vi "Tree Map from Pretty XML.vi"(7 "Parent Path (empty)":string, 10 "Pretty XML":string, 11 "Tree Map In (empty)":T1) -> (0 "Path Invalid":bool, 3 "Tree Map Out":T1)   [LabVIEW 2020, in "Tree Map.lvlib"]
doc: "Unflattens an XML string following the Tree Map API definition. This VI does not work with standard inbuilt LabVIEW XML Flattened Map data.\n\nA starting parent path can be provided if the XML should be unflattened as a child of a parent already exising in the Tree Map.\n\nReturned error can signify that either the path reconstructed from XML is invalid or a construction of a Tree with the same name was attempted. Node paths need to be unique using this API.\n\n<b>Author:</b> Piotr Kruczkowski <PrimaryKey>\n<b>License:</b> NewBSD\n\nCopyright (c) 2019, National Instruments\nAll rights reserved.\n\nRedistribution and use in source and binary forms, with or without\nmodification, are permitted provided that the following conditions are met:\n1. Redistributions of source code must retain the above copyright\n notice, this list of conditions and the following disclaimer.\n2. Redistributions in binary form must reproduce the above copyright\n notice, this list of conditions and the following disclaimer in the\n documentation and/or other materials provided with the distribution.\n3. Neither the name of National Instruments nor the\n names of its contributors may be used to endorse or promote products\n derived from this software without specific prior written permission.\n\nTHIS SOFTWARE IS PROVIDED BY National Instruments ''AS IS'' AND ANY\nEXPRESS OR IMPLIED WARRANTIES, INCLUDING, BUT NOT LIMITED TO, THE IMPLIED\nWARRANTIES OF MERCHANTABILITY AND FITNESS FOR A PARTICULAR PURPOSE ARE\nDISCLAIMED. IN NO EVENT SHALL National Instruments BE LIABLE FOR ANY\nDIRECT, INDIRECT, INCIDENTAL, SPECIAL, EXEMPLARY, OR CONSEQUENTIAL DAMAGES\n(INCLUDING, BUT NOT LIMITED TO, PROCUREMENT OF SUBSTITUTE GOODS OR SERVICES;\nLOSS OF USE, DATA, OR PROFITS; OR BUSINESS INTERRUPTION) HOWEVER CAUSED AND\nON ANY THEORY OF LIABILITY, WHETHER IN CONTRACT, STRICT LIABILITY, OR TORT\n(INCLUDING NEGLIGENCE OR OTHERWISE) ARISING IN ANY WAY OUT OF THE USE OF THIS\nSOFTWARE, EVEN IF ADVISED OF THE POSSIBILITY OF SUCH DAMAGE."
uses:
  Tree Map.lvlib
  Tree Map Data.ctl
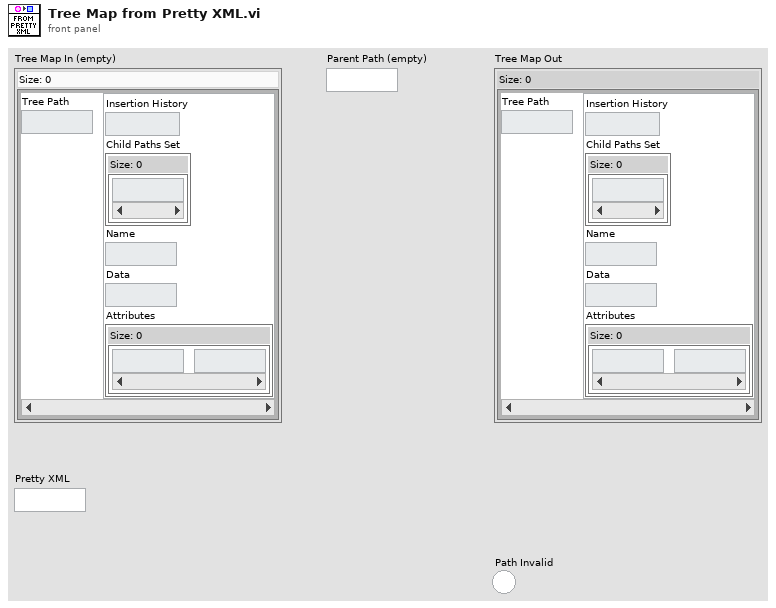
[diagram p1: front panel]
types:
  T1 = typedef "Tree Map.lvlib/Tree Map Data.ctl" = map{string, cluster{"Insertion History":i32, "Child Paths Set":set{string}, "Name":string, "Data":string, "Attributes":map{string, string}}}
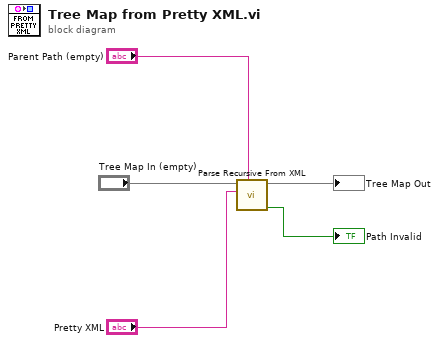
[diagram p0: block diagram]
diagram:
  n1 = call "Parse Recursive From XML.vi"("Parent Path (empty)"="Parent Path (empty)", "XML String"="Pretty XML", "Tree Map In"="Tree Map In (empty)") -> ("Path Invalid"=→"Path Invalid":bool, "Tree Map Out"=→"Tree Map Out":T1)  [unwired: 6 in, 1 out]
